vi "myRIO_BRig_RT_dataExp_ENL_min.vi"() -> (2 "output_ENL_min":i32)   [LabVIEW 2014]
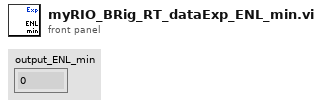
[diagram p1: front panel]
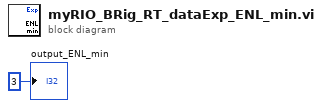
[diagram p0: block diagram]
diagram:
  "output_ENL_min" <- 3 ("output_iBlock")
